vi "Untitled 1.vi"() -> ()   [LabVIEW 2020]
panel:
  in  "module path":path
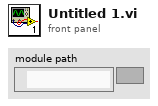
[diagram p1: front panel]
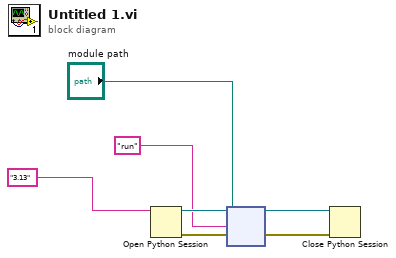
[diagram p0: block diagram]
diagram:
  n1 = Open Python Session(python version="3.13" ("Python version")) -> (session out=w7:refnum<k35>, error out=w5:errorcluster)  [unwired: 2 in]
  n2 = node(w7, "module path", "run" ("function name"), w5) -> (w6:refnum<k35>, w4:errorcluster)  [unwired: 2 in, 2 out]
  n3 = Close Python Session(session in=w6, error in=w4) -> ()  [unwired: 1 out]
